vi "rate_limit.vi"(1 "Rate Limit":dbl, 2 "In":dbl) -> (0 "Out":dbl)   [LabVIEW 2023]
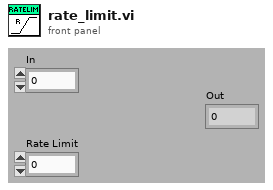
[diagram p1: front panel]
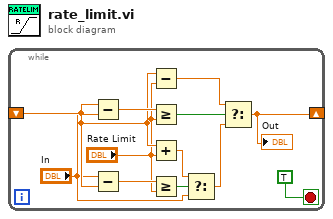
[diagram p0: block diagram]
diagram:
  n1 = while {
    shift-right: [w2] -> _
    shift-left: _ -> [w5]
    stop <- TRUE stop-if-true
    n2 = Subtract(x=w5, y="In") -> (x-y=w8:dbl)
    n3 = Subtract(x="In", y=w5) -> (x-y=w11:dbl)
    n4 = Subtract(x=w5, y="Rate Limit") -> (x-y=w3:dbl)
    n5 = Greater Or Equal?(x=w8, y="Rate Limit") -> (x >= y?=w7:bool)
    n6 = Add(x=w5, y="Rate Limit") -> (x+y=w9:dbl)
    n7 = Greater Or Equal?(x=w11, y="Rate Limit") -> (x >= y?=w10:bool)
    n8 = Select(t=w9, s=w10, f="In") -> (s? t:f=w6:dbl)
    n9 = Select(t=w3, s=w7, f=w6) -> (s? t:f=w2:dbl)
    "Out" <- w2
  }
